vi "Coordenadas espaçadores.vi"(8 "error in (no error)":errorcluster, 11 "Dados SP":T1={"Condutor"={"Pc (N/m)"=0.0, "Mod.Young (N/m²)"=0.0, "Dil.Term.c (m/°C)"=0.0, "Área  (m²)"=0.0, "Tração EDS (N)"=0.0, "Tração Torig(N)"=0.0, "Tração Talta (N)"=0.0}, "Suporte"={"Ps (N/m)"=0.0, "Es (N/m²)"=0.0, "DTc (1/°C)"=0.0, "Área sup (m²)"=0.0, "Tração EDS sup (N)"=0.0, "Tração AT sup (N)"=0.0, "Flecha sup AT (m)"=0.0}, "Projeto"={"Temp. EDS (°C)"=0.0, "Lim.original (°C)"=0.0, "Lim.extend. (°C)"=0.0, "N. cabo/fase"=1.0}, "Vetor de dados"={"Coor.X.esp"=[], "Coor.Y.Esp."=[], "Sub.vao X"=[], "Sub.vao Y"=[], "CoordY.sup"=[], "CoordX.sup"=[]}, "Subvão"={"N. Esp."=0.0, "F.lim (m)"=0.0, "Ext.calc"=0.0, "Ext.definido"=0.0, "Comp.cabo"=0.0, "Ext.55%"=0.0, "Tração sub\nAT (N)"=0.0, "Ext.sel."=0.0, "Flecha lim.\ncalc (m)"=0.0}, "Vão"={"Extensão (m)"=0.0, "Desnivel (m)"=0.0, "Ext.Lim sub (m)"=0.0, "Flecha à 60 °C"=0.0}} {"Projeto"."N. cabo/fase" min=1.0 max=8.0 step=1.0 format="%#_1f"}) -> (0 "error out":errorcluster, 3 "Dados SP Out":T1={"Condutor"={"Pc (N/m)"=0.0, "Mod.Young (N/m²)"=0.0, "Dil.Term.c (m/°C)"=0.0, "Área  (m²)"=0.0, "Tração EDS (N)"=0.0, "Tração Torig(N)"=0.0, "Tração Talta (N)"=0.0}, "Suporte"={"Ps (N/m)"=0.0, "Es (N/m²)"=0.0, "DTc (1/°C)"=0.0, "Área sup (m²)"=0.0, "Tração EDS sup (N)"=0.0, "Tração AT sup (N)"=0.0, "Flecha sup AT (m)"=0.0}, "Projeto"={"Temp. EDS (°C)"=0.0, "Lim.original (°C)"=0.0, "Lim.extend. (°C)"=0.0, "N. cabo/fase"=1.0}, "Vetor de dados"={"Coor.X.esp"=[], "Coor.Y.Esp."=[], "Sub.vao X"=[], "Sub.vao Y"=[], "CoordY.sup"=[], "CoordX.sup"=[]}, "Subvão"={"N. Esp."=0.0, "F.lim (m)"=0.0, "Ext.calc"=0.0, "Ext.definido"=0.0, "Comp.cabo"=0.0, "Ext.55%"=0.0, "Tração sub\nAT (N)"=0.0, "Ext.sel."=0.0, "Flecha lim.\ncalc (m)"=0.0}, "Vão"={"Extensão (m)"=0.0, "Desnivel (m)"=0.0, "Ext.Lim sub (m)"=0.0, "Flecha à 60 °C"=0.0}} {"Projeto"."N. cabo/fase" min=1.0 max=8.0 step=1.0 format="%#_1f"}, 5 "CoordXY.Esp":cluster{dbl[], dbl[]})   [LabVIEW 2020]
uses:
  controles/SP data.ctl
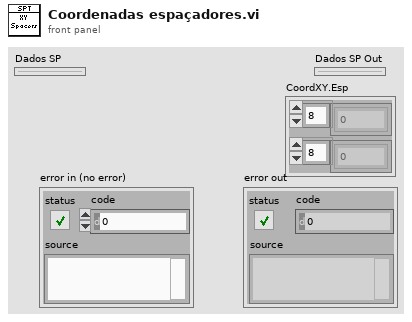
[diagram p1: front panel]
types:
  T1 = typedef "SP data.ctl" = cluster{"Condutor":cluster{"Pc (N/m)":dbl, "Mod.Young (N/m²)":dbl, "Dil.Term.c (m/°C)":dbl, "Área  (m²)":dbl, "Tração EDS (N)":dbl, "Tração Torig(N)":dbl, "Tração Talta (N)":dbl}, "Suporte":cluster{"Ps (N/m)":dbl, "Es (N/m²)":dbl, "DTc (1/°C)":dbl, "Área sup (m²)":dbl, "Tração EDS sup (N)":dbl, "Tração AT sup (N)":dbl, "Flecha sup AT (m)":dbl}, "Projeto":cluster{"Temp. EDS (°C)":dbl, "Lim.original (°C)":dbl, "Lim.extend. (°C)":dbl, "N. cabo/fase":dbl}, "Vetor de dados":cluster{"Coor.X.esp":dbl[], "Coor.Y.Esp.":dbl[], "Sub.vao X":dbl[], "Sub.vao Y":dbl[], "CoordY.sup":dbl[], "CoordX.sup":dbl[]}, "Subvão":cluster{"N. Esp.":dbl, "F.lim (m)":dbl, "Ext.calc":dbl, "Ext.definido":dbl, "Comp.cabo":dbl, "Ext.55%":dbl, "Tração sub\nAT (N)":dbl, "Ext.sel.":dbl, "Flecha lim.\ncalc (m)":dbl}, "Vão":cluster{"Extensão (m)":dbl, "Desnivel (m)":dbl, "Ext.Lim sub (m)":dbl, "Flecha à 60 °C":dbl}}
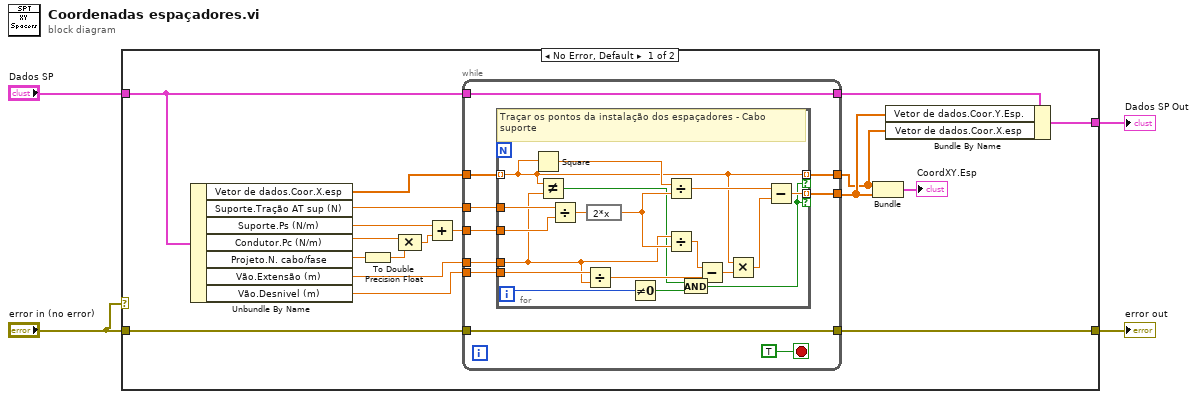
[diagram p0: block diagram]
diagram:
  n1 = case shown="No Error, Default" "error in (no error)" {
    tunnel: [w21 w51] -> w4
    tunnel: "Dados SP" -> [w8 w52]
    tunnel: "error in (no error)" -> [w7 w51]
    tunnel: [w6 w52] -> w2
    frame No Error {
      n2 = Unbundle By Name(w8) -> ("Vetor de dados.Coor.X.esp"=w11:dbl[], "Suporte.Tração AT sup (N)"=w20:dbl, "Suporte.Ps (N/m)"=w19:dbl, "Condutor.Pc (N/m)"=w17:dbl, "Projeto.N. cabo/fase"=w13:dbl, "Vão.Extensão (m)"=w14:dbl, "Vão.Desnivel (m)"=w18:dbl)
      n3 = To Double Precision Float(number=w13) -> (double precision float=w12:dbl)
      n4 = Compound Arithmetic op=MULTIPLY(w17, w12) -> (w15:dbl)
      n5 = Add(x=w19, y=w15) -> (x+y=w16:dbl)
      n6 = while {
        tunnel: w14 -> [w32]
        tunnel: [w31] -> w5
        tunnel: [w30] -> w9
        tunnel: w11 -> [w29]
        tunnel: w20 -> [w28]
        tunnel: w16 -> [w27]
        tunnel: w8 -> [w25]
        tunnel: [w25] -> w10
        tunnel: w7 -> [w24]
        tunnel: [w24] -> w21
        tunnel: w18 -> [w23]
        stop <- TRUE stop-if-true
        n7 = for {
          tunnel: [w42] -> w30 mode=indexing if=w34
          tunnel: w29 -> [w36] mode=indexing
          tunnel: [w36] -> w31 mode=indexing if=w34
          tunnel: w32 -> [w35]
          tunnel: w28 -> [w41]
          tunnel: w27 -> [w40]
          tunnel: w23 -> [w39]
          i -> [w38]
          # "Traçar os pontos da instalação dos espaçadores - Cabo suporte"
          n8 = Square(x=w36) -> (x^2=w44:dbl)
          n9 = Not Equal?(x=w36, y=w35) -> (x != y?=w33:bool)
          n10 = Divide(x=w41, y=w40) -> (x/y=w50:dbl)
          n11 = Divide(x=w39, y=w35) -> (x/y=w48:dbl)
          n12 = expression code="2*x"(w50) -> (w45:dbl)
          n13 = Not Equal To 0?(x=w38) -> (x != 0?=w37:bool)
          n14 = Divide(x=w44, y=w45) -> (x/y=w43:dbl)
          n15 = Divide(x=w35, y=w45) -> (x/y=w49:dbl)
          n16 = And(x=w33, y=w37) -> (x .and. y?=w34:bool)
          n17 = Subtract(x=w49, y=w48) -> (x-y=w47:dbl)
          n18 = Multiply(x=w36, y=w47) -> (x*y=w46:dbl)
          n19 = Subtract(x=w43, y=w46) -> (x-y=w42:dbl)
        }
      }
      n20 = Bundle(w5, w9) -> (→"CoordXY.Esp":cluster{dbl[], dbl[]})  [unwired: 1 in]
      n21 = Bundle By Name(cluster=w10, "Vetor de dados.Coor.Y.Esp."=w9, "Vetor de dados.Coor.X.esp"=w5) -> (w6:T1)
    }
    frame Error {
    }
  }
  "Dados SP Out" <- w2
  "error out" <- w4
